vi "Set Flow.vi"(8 "error in":errorcluster, 10 "High Flow?":bool, 11 "TSI 3025 in":refnum<class "TSI 3025.lvclass">) -> (0 "error out":errorcluster, 3 "TSI 3025 out":refnum<class "TSI 3025.lvclass">)   [LabVIEW 2014, in "TSI 3025.lvclass"]
uses:
  TSI 3025.lvclass
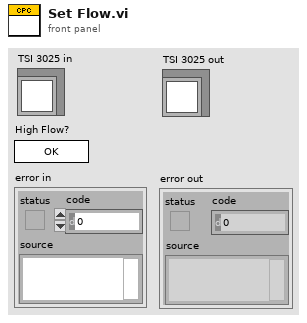
[diagram p1: front panel]
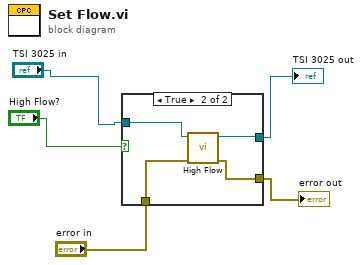
[diagram p0: block diagram]
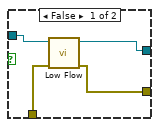
[diagram p2: hidden frame]
diagram:
  n1 = case shown="True" "High Flow?" {
    tunnel: "TSI 3025 in" -> [w9 w13]
    tunnel: [w8 w12] -> w4
    tunnel: "error in" -> [w7 w11]
    tunnel: [w6 w10] -> w1
    frame False {
      n2 = call "Low Flow.vi"("error in"=w7, "TSI 3025 in"=w9) -> ("error out"=w6:errorcluster, "TSI 3025 out"=w8:refnum<class "TSI 3025.lvclass">)  [unwired: 7 in, 1 out]
    }
    frame True {
      n3 = call "High Flow.vi"("error in"=w11, "TSI 3025 in"=w13) -> ("error out"=w10:errorcluster, "TSI 3025 out"=w12:refnum<class "TSI 3025.lvclass">)  [unwired: 7 in, 1 out]
    }
  }
  "error out" <- w1
  "TSI 3025 out" <- w4
